vi "XCP and CCP - Field Table Control.vi"() -> ()   [LabVIEW 2011]
doc: "Sample numeric display item."
uses:
  <vilib>/NI Veristand/Display Template Support/Display Template Support.llb/cluster_Screen Item Settings.ctl
  <vilib>/NI Veristand/Display Template Support/Display Template Support.llb/cluster_Graph Scale Settings.ctl
  <vilib>/NI Veristand/Display Template Support/Display Template Support.llb/cluster_Graph Plot Settings.ctl
  Tables/XCPCCP TBL2D.xctl
  NationalInstruments.VeriStand.SystemStorage
  Controls/Control Links.ctl
  Controls/ECUMC Item.ctl
  <vilib>/NI Veristand/Display Template Support/Display Template Support.llb/enum_Display Template Handler Minimal To Widget Msg.ctl
  <vilib>/NI Veristand/Display Template Support/Display Template Support.llb/enum_Display Template Handler Minimal To Workspace.ctl
  Controls/All Link Data.ctl
  Controls/LinkData.ctl
  <vilib>/ECUMC/NIVS/Support Files.llb/Item Properties.ctl
  <vilib>/ECUMC/NIVS/Support Files.llb/Address Property.ctl
  <vilib>/ECUMC/NIVS/Support Files.llb/Extension Property.ctl
  <vilib>/ECUMC/NIVS/Support Files.llb/Data Type Property.ctl
  <vilib>/ECUMC/NIVS/Support Files.llb/Byte Order Property.ctl
  <vilib>/ECUMC/NIVS/Support Files.llb/Maximum Property.ctl
  <vilib>/ECUMC/NIVS/Support Files.llb/Minimum Property.ctl
  <vilib>/ECUMC/NIVS/Support Files.llb/Read Only Property.ctl
  <vilib>/ECUMC/NIVS/Support Files.llb/Unit Property.ctl
  <vilib>/ECUMC/NIVS/Support Files.llb/Comment Property.ctl
  <vilib>/ECUMC/NIVS/Support Files.llb/X Dimension Property.ctl
  <vilib>/ECUMC/NIVS/Support Files.llb/Y Dimension Property.ctl
  <vilib>/ECUMC/NIVS/Support Files.llb/Is Virtual Property.ctl
  Tables/Limits TBL2D.ctl
  <vilib>/ECUMC/NIVS/Support Files.llb/Item Type.ctl
  SubVIs/Get Conn Status Chan Path.vi
  SubVIs/Check Link for Char or Meas.vi
  <vilib>/NI Veristand/Display Template Support/Display Template Support.llb/sub_Display Template Handler Custom.vi
  <vilib>/ECUMC/NIVS/Set Char Data.vi
  <vilib>/ECUMC/NIVS/Support Files.llb/Set Char Data (2d, TCP).vi
  <vilib>/NI Veristand/Execution/Workspace/NI VeriStand - Set Channel Value.vi
  <vilib>/NI Veristand/Execution/Workspace/NI VeriStand - Set Multiple Channel Values.vi
  <vilib>/NI Veristand/Execution/Workspace/NI VeriStand - Get Channel Value.vi
  <vilib>/NI Veristand/Execution/Workspace/NI VeriStand - Get Multiple Channel Values.vi
  <vilib>/NI Veristand/Execution/Workspace/NI VeriStand - Get System State.vi
  <vilib>/ECUMC/NIVS/Support Files.llb/Get Single Char Properties (TCP).vi
  <vilib>/ECUMC/NIVS/Get Char Data.vi
  <vilib>/ECUMC/NIVS/Support Files.llb/Get Single Char Data (TCP).vi
  <vilib>/ECUMC/NIVS/Get Meas Data.vi
  <vilib>/ECUMC/NIVS/Support Files.llb/Get Single Meas Data (TCP).vi
  <vilib>/NI Veristand/Execution/Workspace/NI VeriStand - Get Single Channel Value.vi
  <vilib>/NI Veristand/Execution/Workspace/NI_VS Workspace ExecutionAPI.lvlib
  <vilib>/ECUMC/NIVS/XCPCCP Add-On Execution API.lvlib
  <vilib>/ECUMC/NIVS/Support Files.llb/XCP and CCP Master Custom Device.lvlib
panel:
  in  "Links":T1
  out "Selected Field":string
  in  "NIVS.System Definition Root":refnum<k24>
  in  "TBL2D":cluster{"X":sgl[], "Y":sgl[], "Z":sgl[][]}(xcontrol)
  in  "Item.Data":T3
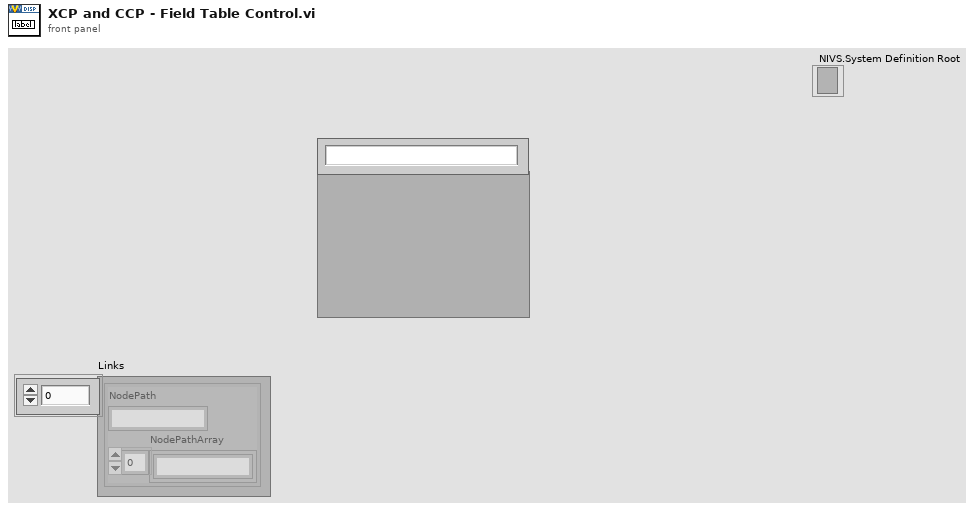
[diagram p1: front panel]
types:
  T1 = typedef "Control Links.ctl" = T2[]
  T2 = typedef "ECUMC Item.ctl" = cluster{"NodePath":string, "NodePathArray":string[]}
  T3 = typedef "cluster_Screen Item Settings.ctl" = cluster{"Template VI":string, "Position X":i32, "Position Y":i32, "Custom":string, "Show Title Bar":bool, "ID":i32, "Always On Top":bool, "Allow Resize":bool, "Allow Minimize":bool, "Allow Close":bool, "Size to Screen":bool, "Screen.ID":i32, "State":enum16{"Normal", "New"}, "Title":string, "Window Bounds":cluster{"[0]":i16, "[1]":i16, "[2]":i16, "[3]":i16}, "Channel Ref":u64, "Unit":string, "Default Units?":bool, "Flash Limit?":bool, "Color 1":u32, "Color 2":u32, "Color 3":u32, "Color 4":u32, "Bck Color":u32, "Fore Color":u32, "Limit 1":dbl, "Limit 2":dbl, "Limit 3":dbl, "Limit 4":dbl, "Limit Mode 1":i32, "Limit Mode 2":i32, "Limit Mode 3":i32, "Limit Mode 4":i32, "Scale Precision":i32, "Scale Min":dbl, "Scale Max":dbl, "Format":i32, "Precision":i32, "Background Type":i32, "IDs":i32[], "Units":string[], "Labels":string[], "Scale Factor":dbl, "Scale Offset":dbl, "YScale Index":u32[], "XScale":T4, "YScales":T4[], "Plots":T5[], "Update Period":dbl, "History Length":dbl, "My.Ref":refnum<vi>, "Is Control?":bool, "Channel Paths":string[], "Custom Data":variant}
  T4 = typedef "cluster_Graph Scale Settings.ctl" = cluster{"Format":u8, "Precision":u8, "Fit":u8, "Label":string, "Use Default Label":bool, "Label Visible":bool, "Min":dbl, "Max":dbl}
  T5 = typedef "cluster_Graph Plot Settings.ctl" = cluster{"Bar Style":u8, "Fill To":i16, "Fill/PtColor":u32, "Line Style":u8, "Line Width":u8, "Color":u32, "Interp":u8, "Point Style":u8}
  T6 = typedef "XCPCCP TBL2D.xctl/Limits TBL2D.ctl" = cluster{"Min X":sgl, "Max X":sgl, "MaxDiff X":sgl, "MaxGrad X":sgl, "Min Y":sgl, "Max Y":sgl, "MaxDiff Y":sgl, "MaxGrad Y":sgl, "Min Z":sgl, "Max Z":sgl, "MaxDiff Z":sgl}
  T7 = typedef "XCP and CCP Master Custom Device.lvlib/Item Properties.ctl" = cluster{"Common":cluster{"Address":T8, "Extension":T9, "Data Type":T10, "Byte Order":T11, "Maximum":T12, "Minimum":T13, "Read Only?":T14, "Unit":T15, "Comment":T16}, "Char Specific":cluster{"X Dimension":T17, "Y Dimension":T18, "char x axis":dbl[], "char y axis":dbl[], "char sizes":u32[]}, "Meas Specific":cluster{"Virtual?":T19}}
  T8 = typedef "XCP and CCP Master Custom Device.lvlib/Address Property.ctl" = u32
  T9 = typedef "XCP and CCP Master Custom Device.lvlib/Extension Property.ctl" = u8
  T10 = typedef "XCP and CCP Master Custom Device.lvlib/Data Type Property.ctl" = enum16{"UBYTE", "SBYTE", "UWORD", "SWORD", "ULONG", "SLONG", "FLOAT32_IEEE", "FLOAT64_IEEE"}
  T11 = typedef "XCP and CCP Master Custom Device.lvlib/Byte Order Property.ctl" = enum16{"Intel", "Motorola"}
  T12 = typedef "XCP and CCP Master Custom Device.lvlib/Maximum Property.ctl" = dbl
  T13 = typedef "XCP and CCP Master Custom Device.lvlib/Minimum Property.ctl" = dbl
  T14 = typedef "XCP and CCP Master Custom Device.lvlib/Read Only Property.ctl" = bool
  T15 = typedef "XCP and CCP Master Custom Device.lvlib/Unit Property.ctl" = string
  T16 = typedef "XCP and CCP Master Custom Device.lvlib/Comment Property.ctl" = string
  T17 = typedef "XCP and CCP Master Custom Device.lvlib/X Dimension Property.ctl" = u32
  T18 = typedef "XCP and CCP Master Custom Device.lvlib/Y Dimension Property.ctl" = u32
  T19 = typedef "XCP and CCP Master Custom Device.lvlib/Is Virtual Property.ctl" = bool
  T20 = typedef "All Link Data.ctl" = T21[]
  T21 = typedef "LinkData.ctl" = cluster{"Chns":string[], "InSys?":bool, "IP":string, "Port":u16}
  T22 = typedef "enum_Display Template Handler Minimal To Workspace.ctl" = cluster{"Operation":enum16{"SetCustomData", "DeleteItem"}, "Data":variant}
  T23 = typedef "enum_Display Template Handler Minimal To Widget Msg.ctl" = enum16{"Stop", "LaunchConfigDialog"}
  T24 = typedef "NI_VS Workspace ExecutionAPI.lvlib/WorkspaceAPI.ctl" = refnum<k24>
  T25 = typedef "NI_VS Workspace ExecutionAPI.lvlib/SystemStateEventRef.ctl" = cluster{"CustDatRef":refnum<user-event>, "EvtRef":refnum<k27>}
  T26 = typedef "NI_VS Workspace ExecutionAPI.lvlib/SystemStateRegEventRef.ctl" = refnum<event-registration>
  T27 = cluster{"Event Registration Refnum":refnum<event-registration>, "SystemChangeEventRef":T26}
  T28 = typedef "XCP and CCP Master Custom Device.lvlib/Item Type.ctl" = enum16{"Scalar Characteristic", "Curve Characteristic", "Field Characteristic", "Measurement"}
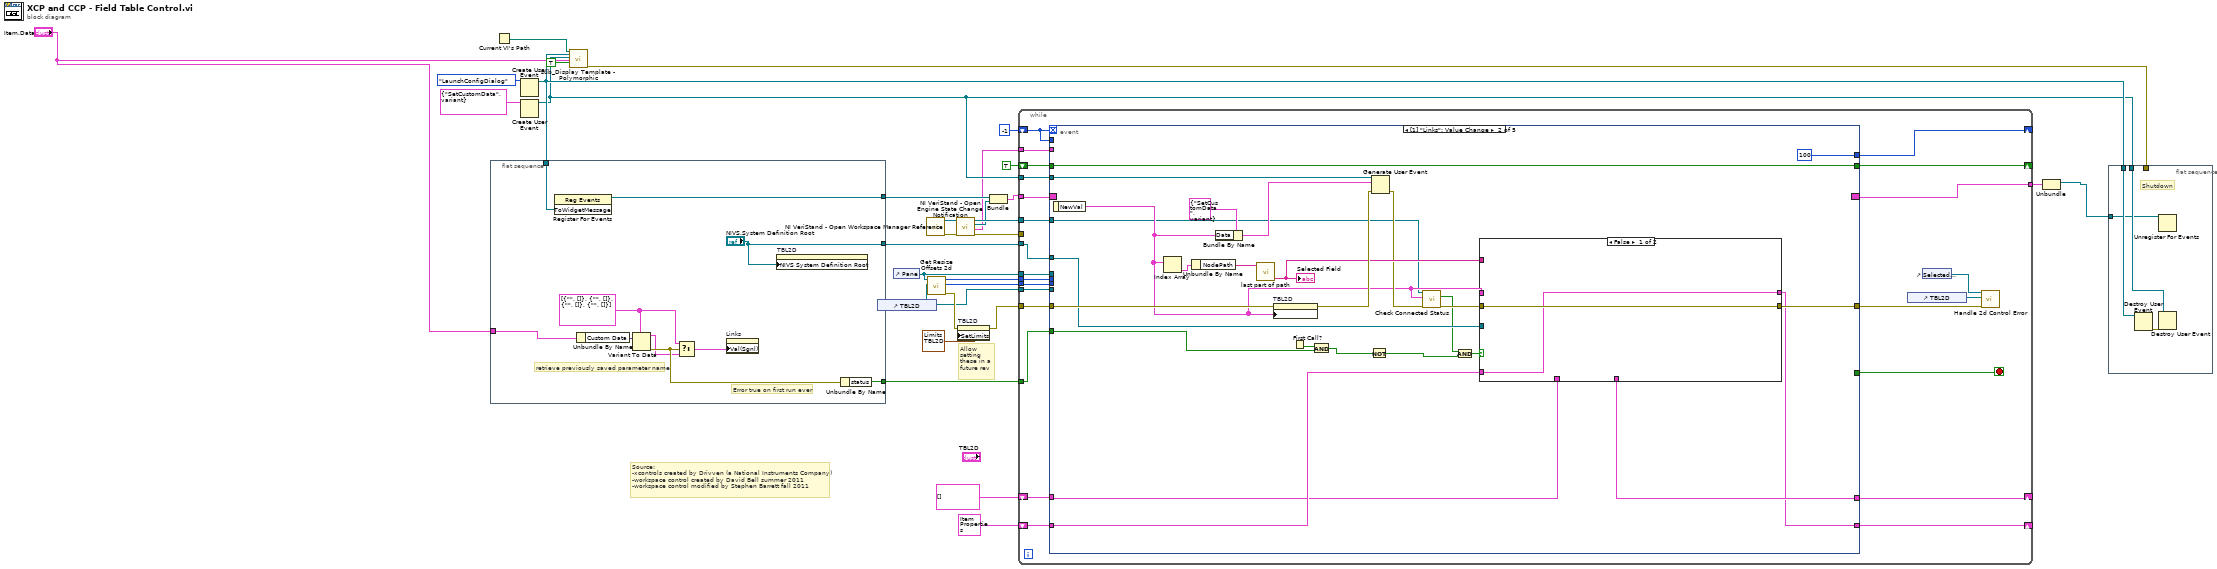
[diagram p0: block diagram]
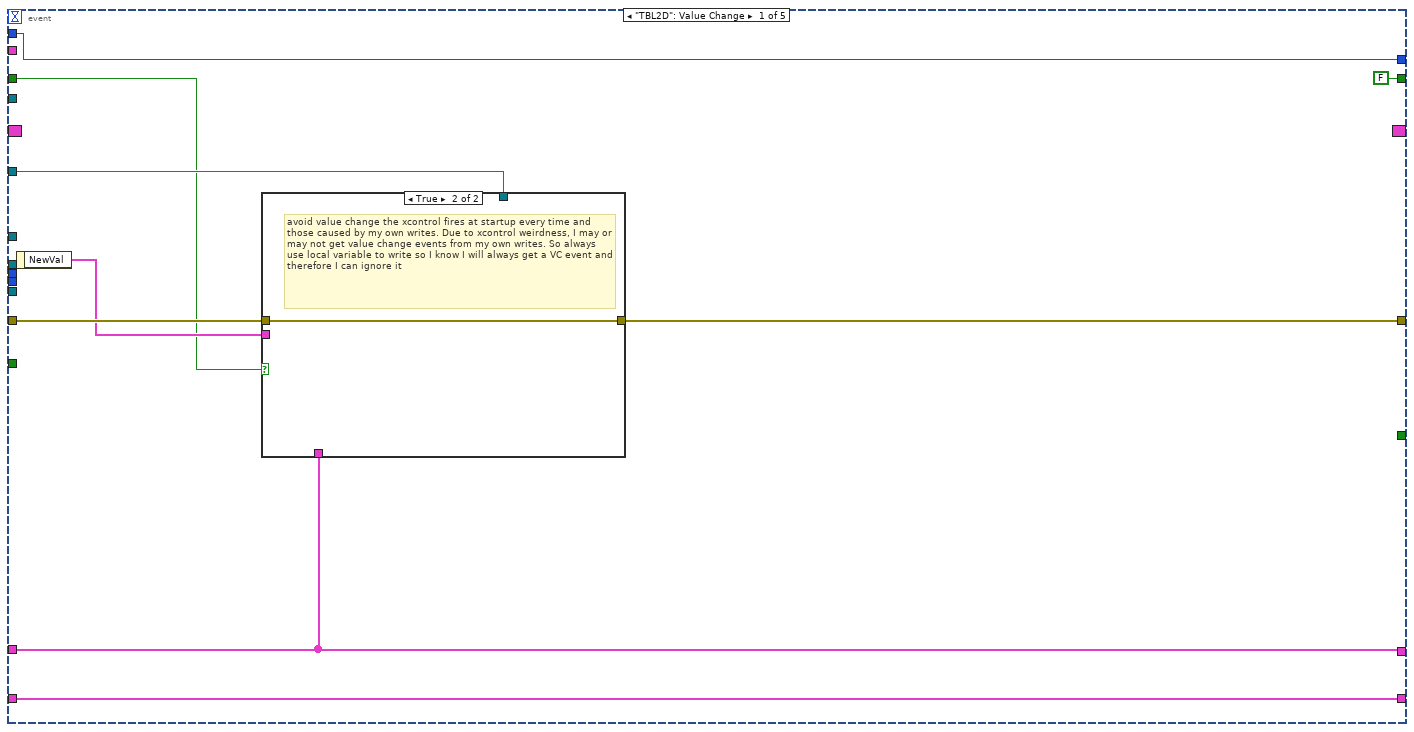
[diagram p2: hidden frame]
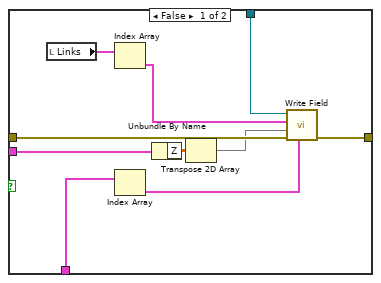
[diagram p3: hidden frame]
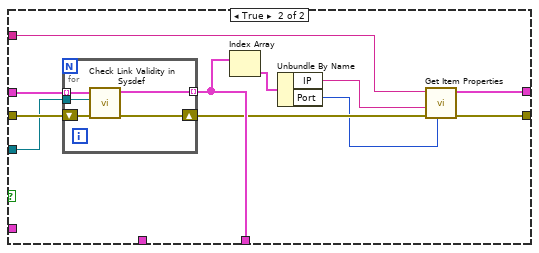
[diagram p4: hidden frame]
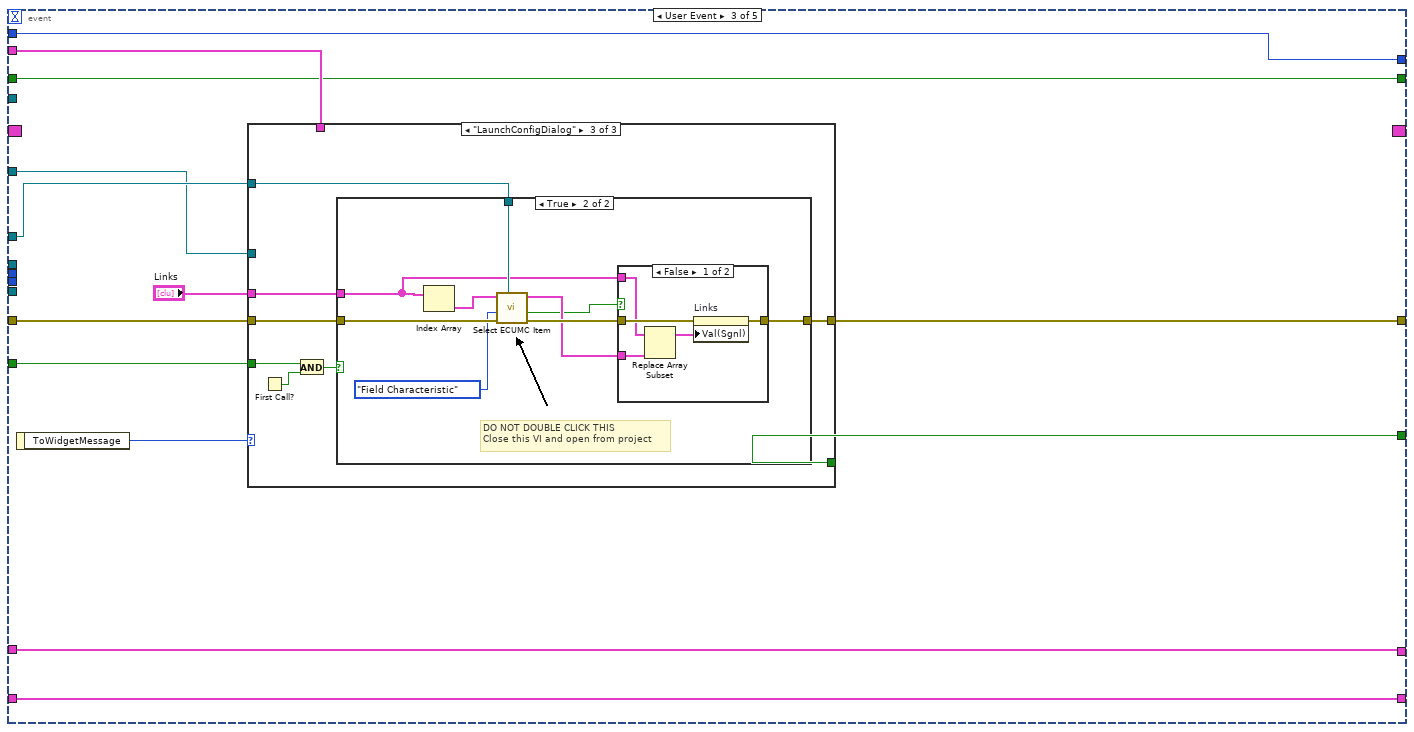
[diagram p5: hidden frame]
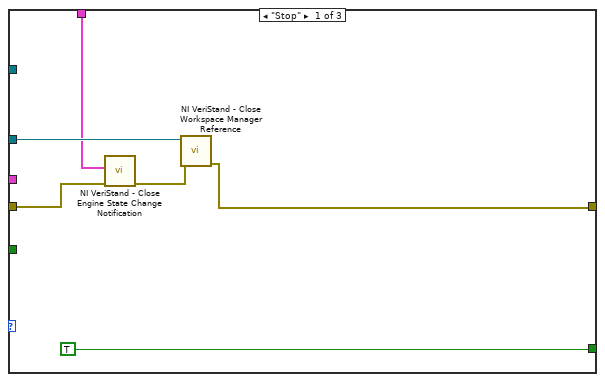
[diagram p6: hidden frame]
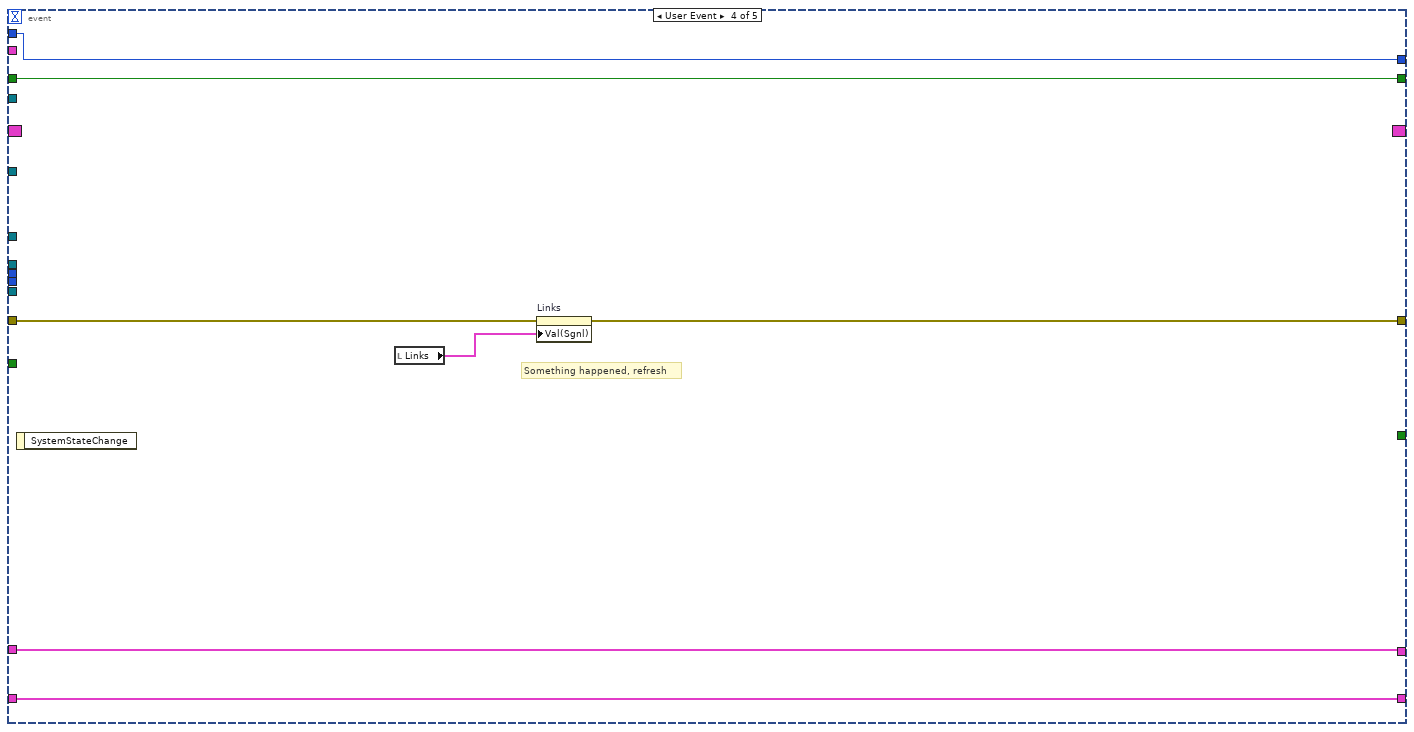
[diagram p10: hidden frame]
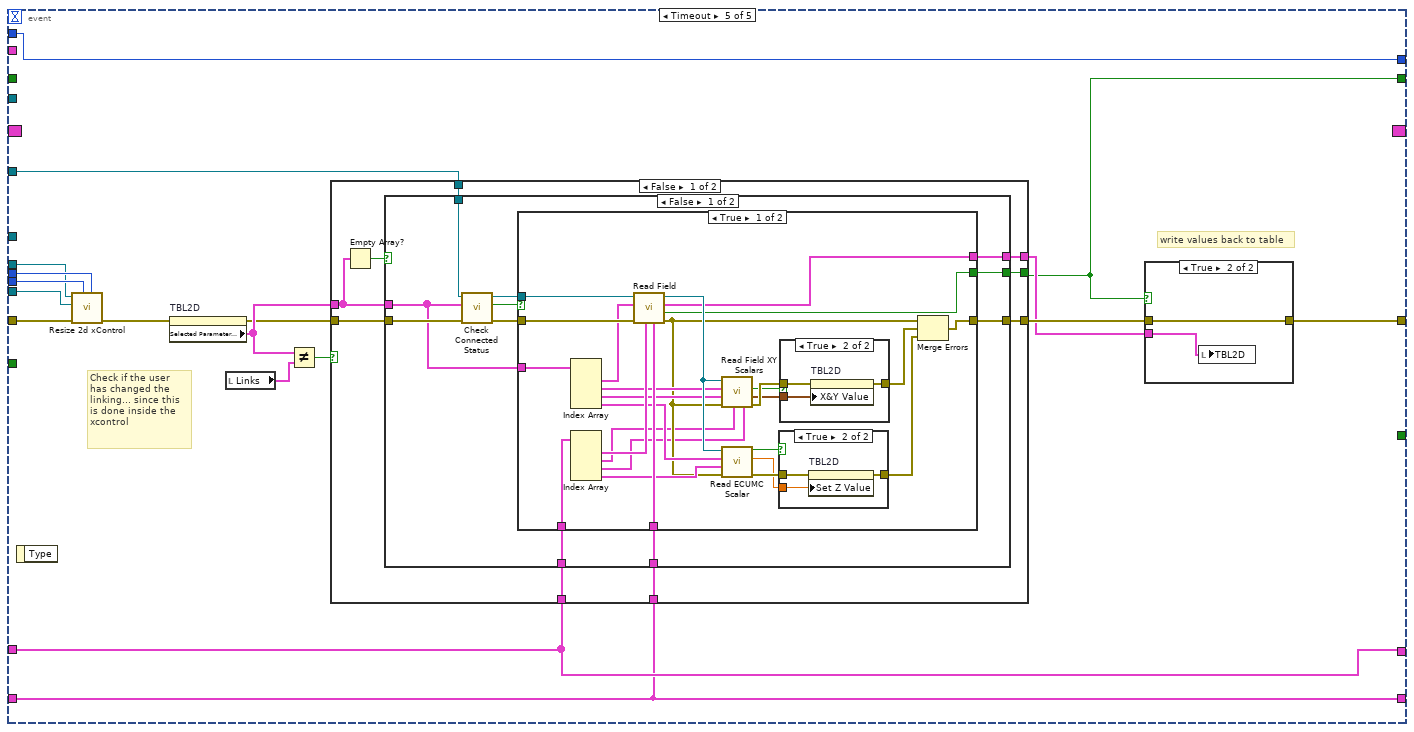
[diagram p11: hidden frame]
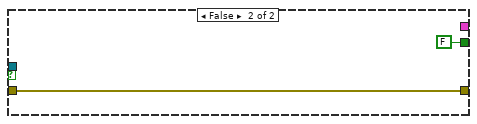
[diagram p15: hidden frame]
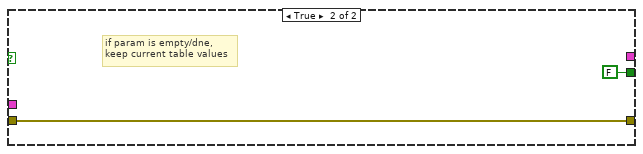
[diagram p16: hidden frame]
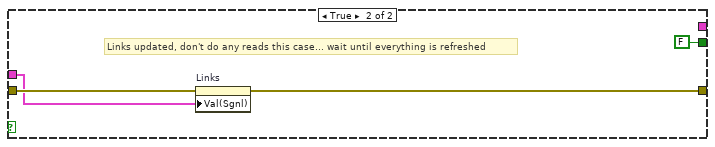
[diagram p17: hidden frame]
diagram:
  # "Source: \n-xcontrols created by Drivven (a National Instruments Company)\n-workspace control created by David Bell summer 2011\n-workspace control modified by Stephen Barrett fall 2011"
  # "Allow setting these in a future rev"
  n1 = flat-sequence {
    tunnel: [w41] -> w10
    tunnel: w29 -> [w40]
    tunnel: "Item.Data" -> [w38]
    tunnel: ["NIVS.System Definition Root"] -> w23
    tunnel: [w35] -> w22
    frame #0 {
      w32 = T1 [{"NodePath"="", "NodePathArray"=[]}, {"NodePath"="", "NodePathArray"=[]}, {"NodePath"="", "NodePathArray"=[]}, {"NodePath"="", "NodePathArray"=[]}] ("Links")
      # "Error true on first run ever"
      # "retrieve previously saved parameter name"
      n2 = register-events(w40) -> (reference out=w41:refnum<event-registration>)  [unwired: 2 in, 1 out]
      n3 = Unbundle By Name(w38) -> ("Custom Data"=w39:variant)
      n4 = Variant To Data(type=w32, Variant=w39) -> (data=w33:T1, error out=w36:errorcluster)  [unwired: 1 in]
      n5 = Select(t=w32, s=w36, f=w33) -> (s? t:f=w34:T1)
      n6 = property on="Links" class="Arr (strict)"("Val(Sgnl)"=w34) -> ()  [unwired: 2 in, 2 out]
      n7 = property on="TBL2D" class="XCPCCP TBL2D (strict)"("NIVS System Definition Root"="NIVS.System Definition Root") -> ()  [unwired: 2 in, 2 out]
      n8 = Unbundle By Name(w36) -> ("status"=w35:bool)
    }
  }
  n9 = Current VI's Path() -> (path=w27:path)
  n10 = Create User Event(user event datatype=enum_Display_Template_Handler_Minimal_To_Widget_Msg."LaunchConfigDialog" ("ToWidgetMessage")) -> (user event=w29:refnum<user-event>)  [unwired: 1 in, 1 out]
  n11 = Create User Event(user event datatype=T22 {"Operation"=enum."SetCustomData", "Data"=variant} ("Data")) -> (user event=w26:refnum<user-event>)  [unwired: 1 in, 1 out]
  n12 = call-poly <vilib>:"sub_Display Template - Polymorphic.vi"("Parent.Path"=w27, "ToWidgetEvent"=w29, "ToWorkspace"=w26, "Item.Data"="Item.Data", "Resizable"=TRUE) -> ("error out"=w31:errorcluster)  [unwired: 1 in, 13 out]
  n13 = control-ref of="TBL2D"() -> (w16:refnum<vi>)
  n14 = control-ref of="Pane"() -> (w17:refnum<vi>)
  n15 = call <vilib>:"NI VeriStand - Open Workspace Manager Reference.vi"() -> ("error out"=w11:errorcluster, "WorkspaceManager"=w13:T24)  [unwired: 10 in]
  n16 = call "Get Resize Offsets 2d.vi"("TBL2D Refnum"=w16, "Pane in"=w17) -> ("error out"=w20:errorcluster, "Width Offset"=w19:u32, "Height Offset"=w18:u32)  [unwired: 7 in]
  n17 = call <vilib>:"NI VeriStand - Open Engine State Change Notification.vi"("error in (no error)"=w11, "WorkspaceManager in"=w13) -> ("error out"=w9:errorcluster, "SystemStateRefs"=w5:T25, "SystemChangeEventRef"=w8:T26, "WorkspaceManager out"=w12:T24)  [unwired: 6 in]
  n18 = property on="TBL2D" class="XCPCCP TBL2D (strict)"(error in=w20, "SetLimits"=T6 {"Min X"=-inf, "Max X"=inf, "MaxDiff X"=inf, "MaxGrad X"=inf, "Min Y"=-inf, "Max Y"=inf, "MaxDiff Y"=inf, "MaxGrad Y"=inf, "Min Z"=-inf, "Max Z"=inf, "MaxDiff Z"=inf}) -> (error out=w21:errorcluster)  [unwired: 1 in, 1 out]
  n19 = Bundle("Event Registration Refnum"=w10, "SystemChangeEventRef"=w8) -> (w7:T27)  [unwired: 1 in]
  n20 = while {
    tunnel: w7 -> [w65]
    tunnel: [w64] -> w6
    tunnel: w26 -> [w62]
    tunnel: w21 -> [w63]
    tunnel: w12 -> [w61]
    tunnel: w23 -> [w60]
    tunnel: w22 -> [w59]
    tunnel: w19 -> [w58]
    tunnel: w18 -> [w57]
    tunnel: w17 -> [w56]
    tunnel: w16 -> [w55]
    shift-right: [w54] -> _
    shift-left: T20 [] ("All LinkData") -> [w53]
    shift-right: [w52] -> _
    shift-left: T7 {"Common"={"Address"=0, "Extension"=0, "Data Type"=enum."UBYTE", "Byte Order"=enum."Intel", "Maximum"=0.0, "Minimum"=0.0, "Read Only?"=FALSE, "Unit"="", "Comment"=""}, "Char Specific"={"X Dimension"=0, "Y Dimension"=0, "char x axis"=[], "char y axis"=[], "char sizes"=[]}, "Meas Specific"={"Virtual?"=FALSE}} ("Properties") -> [w51]
    tunnel: w9 -> [_]
    tunnel: w5 -> [w46]
    shift-right: [w45] -> _
    shift-left: -1 -> [w44]
    shift-right: [w43] -> _
    shift-left: TRUE -> [w42]
    stop <- w50 stop-if-true
    n21 = event shown="[1] \"Links\": Value Change" {
      selector: w65 -> [_ _ _ _ _]
      dyn-events: [_ _ _ _ _] -> w64
      timeout: w44 -> [_ _ _ _ _]
      tunnel: w63 -> [w73 w106 w142 w178 w196]
      tunnel: w62 -> [_ w107 _ _ _]
      tunnel: [w72 w101 w137 w176 w184] -> w49
      tunnel: w61 -> [w71 w92 w139 _ w198]
      tunnel: [_ _ w138 _ _] -> w50
      tunnel: w60 -> [_ w104 w140 _ _]
      tunnel: w59 -> [_ w99 w141 _ _]
      tunnel: w58 -> [_ _ _ _ w194]
      tunnel: w57 -> [_ _ _ _ w193]
      tunnel: w56 -> [_ _ _ _ w192]
      tunnel: w55 -> [_ _ _ _ w191]
      tunnel: [w70 w103 w136 w180 w189] -> w54
      tunnel: w53 -> [w70 w96 w136 w180 w189]
      tunnel: [w74 w100 w135 w179 w188] -> w52
      tunnel: w51 -> [w74 w97 w135 w179 w188]
      tunnel: w46 -> [_ _ w133 _ _]
      tunnel: [w68 100 w132 w175 w182] -> w45
      tunnel: w44 -> [w68 _ w132 w175 w182]
      tunnel: [FALSE ("Updated") w86 w131 w174 w181] -> w43
      tunnel: w42 -> [w67 w86 w131 w174 _]
      event "TBL2D": Value Change {
        n22 = event-data() -> ("NewVal"=w69:cluster{"X":sgl[], "Y":sgl[], "Z":sgl[][]})  [unwired: 1 in]
        n23 = case shown="True" w67 {
          tunnel: w73 -> [w84 w85]
          tunnel: [w83 w85] -> w72
          tunnel: w71 -> [w82 _]
          tunnel: w70 -> [w81 _]
          tunnel: w69 -> [w80 _]
          frame False {
            n24 = local read "Links"() -> (w79:T1)
            n25 = Index Array(array=w79) -> (element=w78:T2)  [unwired: 1 in]
            n26 = Index Array(array=w81) -> (element=w77:T21)  [unwired: 1 in]
            n27 = Unbundle By Name(w80) -> ("Z"=w76:sgl[][])
            n28 = Transpose 2D Array(2D array=w76) -> (transposed array=w75:sgl[][])
            n29 = call "Write Field.vi"("LinkData"=w77, "Error In"=w84, "Characteristic Field Values"=w75, "Link"=w78, "WorkspaceManager"=w82) -> ("Error Out"=w83:errorcluster)  [unwired: 5 in, 1 out]
          }
          frame True {
            # "avoid value change the xcontrol fires at startup every time and those caused by my own writes. Due to xcontrol weirdness, I may or may not get value change events from my own writes. So always use local variable to write so I know I will always get a VC event and therefore I can ignore it"
          }
        }
      }
      event Value Change {
        n30 = event-data() -> ("NewVal"=w93:T1)  [unwired: 1 in]
        n31 = Index Array(array=w93) -> (element=w111:T2)  [unwired: 1 in]
        n32 = Unbundle By Name(w111) -> ("NodePath"=w105:string)
        n33 = Bundle By Name(cluster=T22 {"Operation"=enum."SetCustomData", "Data"=variant} ("event data"), "Data"=w93) -> (w108:T22)
        n34 = call "last part of path.vi"("String"=w105) -> ("Last Part"=w102:string)  [unwired: 10 in]
        "Selected Field" <- w102
        n35 = property on="TBL2D" class="XCPCCP TBL2D (strict)"(error in=w106, "Selected Parameter 2D"=w93) -> (error out=w110:errorcluster)  [unwired: 1 in, 1 out]
        n36 = First Call?() -> (First Call?: T/F=w98:bool)
        n37 = And(x=w98, y=w99) -> (x .and. y?=w91:bool)
        n38 = Not(x=w91) -> (.not. x?=w90:bool)
        n39 = Generate User Event(user event=w107, event data cluster=w108, error in=w110) -> (error out=w94:errorcluster)  [unwired: 1 out]
        n40 = call "Check Connected Status.vi"("Error In"=w94, "Links"=w93, "WorkspaceManager in"=w92) -> ("Error Out"=w95:errorcluster, "Connected?"=w88:bool)  [unwired: 6 in, 1 out]
        n41 = And(x=w88, y=w90) -> (x .and. y?=w89:bool)
        n42 = case shown="False" w89 {
          tunnel: w95 -> [w114 w125]
          tunnel: w93 -> [_ w124]
          tunnel: w104 -> [_ w123]
          tunnel: [w112 w122] -> w103
          tunnel: w102 -> [_ w120]
          tunnel: [w114 w117] -> w101
          tunnel: [w113 w116] -> w100
          tunnel: w97 -> [w113 _]
          tunnel: w96 -> [w112 _]
          frame False {
          }
          frame True {
            n43 = for {
              shift-right: [w129] -> w121
              shift-left: w125 -> [w130]
              tunnel: w124 -> [w128] mode=indexing
              tunnel: w123 -> [w127]
              tunnel: [w126] -> w122 mode=indexing
              n44 = call "Check Link Validity in Sysdef.vi"("error in (no error)"=w130, "SysDef Root"=w127, "Link"=w128) -> ("error out"=w129:errorcluster, "LinkData"=w126:T21)  [unwired: 7 in]
            }
            n45 = Index Array(array=w122) -> (element=w115:T21)  [unwired: 1 in]
            n46 = Unbundle By Name(w115) -> ("IP"=w119:string, "Port"=w118:u16)
            n47 = call-poly <vilib>:"Get Item Properties.vi"("Port"=w118, "error in (no error)"=w121, "IP or DNS Name"=w119, "Characteristic"=w120) -> ("error out"=w117:errorcluster, "Properties"=w116:T7)  [unwired: 6 in]
          }
        }
      }
      event User Event {
        n48 = event-data() -> ("ToWidgetMessage"=w143:T23)  [unwired: 1 in]
        n49 = case shown="\"LaunchConfigDialog\"" w143 {
          tunnel: [TRUE ("1-D array?") _ _] -> w138
          tunnel: w140 -> [_ _ w157]
          tunnel: w139 -> [w148 _ _]
          tunnel: "Links" -> [_ _ w154]
          tunnel: w142 -> [w146 w150 w156]
          tunnel: [w147 w150 w155] -> w137
          tunnel: w141 -> [_ _ w153]
          tunnel: w133 -> [w144 _ _]
          frame "Stop" {
            n50 = call <vilib>:"NI VeriStand - Close Engine State Change Notification.vi"("error in (no error)"=w146, "SystemStateRefs"=w144) -> ("error out"=w145:errorcluster)  [unwired: 9 in]
            n51 = call <vilib>:"NI VeriStand - Close Workspace Manager Reference.vi"("error in (no error)"=w145, "WorkspaceManager"=w148) -> ("error out"=w147:errorcluster)  [unwired: 9 in]
          }
          frame Default {
          }
          frame "LaunchConfigDialog" {
            n52 = First Call?() -> (First Call?: T/F=w151:bool)
            n53 = And(x=w153, y=w151) -> (x .and. y?=w152:bool)
            n54 = case shown="True" w152 {
              tunnel: w157 -> [_ w164]
              tunnel: w154 -> [_ w159]
              tunnel: w156 -> [w158 w166]
              tunnel: [w158 w167] -> w155
              frame False {
              }
              frame True {
                # "DO NOT DOUBLE CLICK THIS\nClose this VI and open from project"
                n55 = Index Array(array=w159) -> (element=w163:T2)  [unwired: 1 in]
                n56 = call "Select ECUMC Item.vi"("NIVS.System Definition Root"=w164, "error in (no error)"=w166, "Item Type"=Item_Type."Field Characteristic", "Link In"=w163) -> ("error out"=w165:errorcluster, "Canceled?"=w161:bool, "Link Out"=w162:T2)  [unwired: 5 in]
                n57 = case shown="False" w161 {
                  tunnel: w165 -> [w172 w173]
                  tunnel: [w171 w173] -> w167
                  tunnel: w162 -> [w168 _]
                  tunnel: w159 -> [w170 _]
                  frame False {
                    n58 = Replace Array Subset(array=w170, new element=w168) -> (w169:T1)  [unwired: 1 in]
                    n59 = property on="Links" class="Arr (strict)"(error in=w172, "Val(Sgnl)"=w169) -> (error out=w171:errorcluster)  [unwired: 1 in, 1 out]
                  }
                  frame True {
                  }
                }
              }
            }
          }
        }
      }
      event User Event {
        # "Something happened, refresh"
        n60 = event-data() -> ()  [unwired: 1 in, 1 out]
        n61 = local read "Links"() -> (w177:T1)
        n62 = property on="Links" class="Arr (strict)"(error in=w178, "Val(Sgnl)"=w177) -> (error out=w176:errorcluster)  [unwired: 1 in, 1 out]
      }
      event Timeout {
        # "Check if the user has changed the linking... since this is done inside the xcontrol"
        # "write values back to table"
        n63 = event-data() -> ()  [unwired: 1 in, 1 out]
        n64 = call "Resize 2d xControl.vi"("Height Offset"=w193, "Width Offset"=w194, "error in (no error)"=w196, "Control in"=w191, "Pane"=w192) -> ("error out"=w195:errorcluster)  [unwired: 6 in]
        n65 = property on="TBL2D" class="XCPCCP TBL2D (strict)"(error in=w195) -> (error out=w186:errorcluster, "Selected Parameter 2D"=w190:T1)  [unwired: 1 in, 1 out]
        n66 = local read "Links"() -> (w197:T1)
        n67 = Not Equal?(x=w190, y=w197) -> (x != y?=w187:bool)
        n68 = case shown="False" w187 {
          tunnel: [w210 w261] -> w185
          tunnel: w198 -> [w209 _]
          tunnel: [w208 _] -> w183
          tunnel: w190 -> [w204 w262]
          tunnel: w189 -> [w207 _]
          tunnel: w188 -> [w206 _]
          tunnel: w186 -> [w205 w263]
          tunnel: [w202 FALSE ("Updated")] -> w181
          frame False {
            n69 = Empty Array?(array=w204) -> (empty?=w203:bool)
            n70 = case shown="False" w203 {
              tunnel: [w221 w259] -> w210
              tunnel: [w220 _] -> w208
              tunnel: w205 -> [w219 w259]
              tunnel: w204 -> [w212 _]
              tunnel: w209 -> [w217 _]
              tunnel: w207 -> [w214 _]
              tunnel: w206 -> [w213 _]
              tunnel: [w211 FALSE ("Updated")] -> w202
              frame False {
                n71 = call "Check Connected Status.vi"("Error In"=w219, "Links"=w212, "WorkspaceManager in"=w217) -> ("Error Out"=w218:errorcluster, "Connected?"=w215:bool, "WorkspaceManager out"=w216:T24)  [unwired: 6 in]
                n72 = case shown="True" w215 {
                  tunnel: [w223 _] -> w220
                  tunnel: w218 -> [w245 w257]
                  tunnel: [w246 w257] -> w221
                  tunnel: w212 -> [w247 _]
                  tunnel: w216 -> [w244 _]
                  tunnel: w214 -> [w242 _]
                  tunnel: w213 -> [w240 _]
                  tunnel: [w222 FALSE ("Updated")] -> w211
                  frame True {
                    n73 = Index Array(array=w247) -> (element #1=w243:T2, element #2=w231:T2, element #3=w230:T2, element #4=w235:T2)  [unwired: 4 in]
                    n74 = Index Array(array=w242) -> (element #1=w241:T21, element #2=w225:T21, element #3=w224:T21, element #4=w236:T21)  [unwired: 4 in]
                    n75 = call "Read Field.vi"("Properties"=w240, "LinkData"=w241, "Error In"=w245, "Link"=w243, "WorkspaceManager"=w244) -> ("Error Out"=w229:errorcluster, "NewVal"=w222:bool, "Table"=w223:cluster{"X":sgl[], "Y":sgl[], "Z":sgl[][]}, "WorkspaceManager out"=w232:T24)  [unwired: 3 in]
                    n76 = call "Read Field XY Scalars.vi"("YLinkData"=w224, "XLinkData"=w225, "Error In"=w229, "YLink"=w230, "XLink"=w231, "WorkspaceManager"=w232) -> ("Error Out"=w228:errorcluster, "Values"=w227:cluster{"Values[0]":dbl, "Values[1]":dbl}, "Changed?"=w226:bool)  [unwired: 3 in]
                    n77 = call "Read ECUMC Scalar.vi"("Error In"=w229, "LinkData"=w236, "Link"=w235, "WorkspaceManager"=w232) -> ("Error Out"=w237:errorcluster, "Value"=w234:dbl, "Changed?"=w233:bool)  [unwired: 5 in]
                    n78 = case shown="True" w233 {
                      tunnel: w237 -> [w248 w251]
                      tunnel: [w248 w250] -> w238
                      tunnel: w234 -> [_ w249]
                      frame False {
                      }
                      frame True {
                        n79 = property on="TBL2D" class="XCPCCP TBL2D (strict)"(error in=w251, "Set Z Value"=w249) -> (error out=w250:errorcluster)  [unwired: 1 in, 1 out]
                      }
                    }
                    n80 = case shown="True" w226 {
                      tunnel: w228 -> [w252 w255]
                      tunnel: [w252 w254] -> w239
                      tunnel: w227 -> [_ w253]
                      frame False {
                      }
                      frame True {
                        n81 = property on="TBL2D" class="XCPCCP TBL2D (strict)"(error in=w255, "X&Y Value"=w253) -> (error out=w254:errorcluster)  [unwired: 1 in, 1 out]
                      }
                    }
                    n82 = Merge Errors(w229, w239, w238) -> (w246:errorcluster)
                  }
                  frame False {
                  }
                }
              }
              frame True {
                # "if param is empty/dne,\nkeep current table values"
              }
            }
          }
          frame True {
            # "Links updated, don't do any reads this case... wait until everything is refreshed"
            n83 = property on="Links" class="Arr (strict)"(error in=w263, "Val(Sgnl)"=w262) -> (error out=w261:errorcluster)  [unwired: 1 in, 1 out]
          }
        }
        n84 = case shown="True" w181 {
          tunnel: w185 -> [w199 w201]
          tunnel: [w199 w201] -> w184
          tunnel: w183 -> [_ w200]
          frame False {
          }
          frame True {
            n85 = local write "TBL2D"(w200) -> ()
          }
        }
      }
    }
    n86 = control-ref of="TBL2D"() -> (w48:refnum<vi>)
    n87 = control-ref of="Selected Field"() -> (w47:refnum<vi>)
    n88 = call "Handle 2d Control Error.vi"("Error In"=w49, "TBL2D Refnum"=w48, "Label"=w47) -> ()  [unwired: 9 in]
  }
  n89 = Unbundle(w6) -> ("Event Registration Refnum"=w3:refnum<event-registration>)  [unwired: 1 out]
  n90 = flat-sequence {
    tunnel: w31 -> [_]
    tunnel: w29 -> [w267]
    tunnel: w26 -> [w265]
    tunnel: w3 -> [w264]
    frame #0 {
      # "Shutdown"
      n91 = Destroy User Event(user event=w267) -> (error out=w266:errorcluster)  [unwired: 1 in]
      n92 = Unregister For Events(event registration refnum=w264) -> ()  [unwired: 1 in, 1 out]
      n93 = Destroy User Event(user event=w265, error in=w266) -> ()  [unwired: 1 out]
    }
  }
